vi "Test Base Card Passthrough(Register).vi"(4 "Iterations":u32=50 min=1 max=64, 11 "device":refnum<k21>="SET-2010-Mod2") -> (0 "error out":errorcluster, 1 "Disconnect Timing":T1, 2 "Connect Timing":T1)   [LabVIEW 2020, in "slsc-switch-benchmarks.lvlib"]
uses:
  slsc-switch-benchmarks.lvlib
  Timing Statistics.ctl
  <vilib>/SLSC/Write Register (U64).vi
  <vilib>/SLSC/Initialize Session with Devices.vi
  <vilib>/SLSC/Close Session.vi
  <vilib>/SLSC/SLSC.lvlib
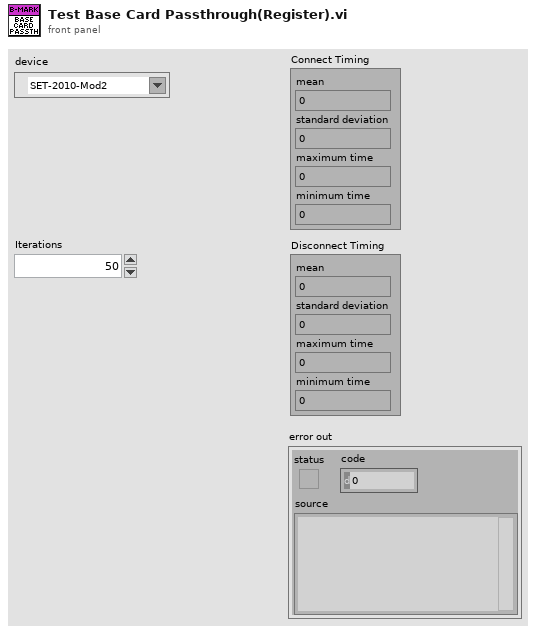
[diagram p1: front panel]
types:
  T1 = typedef "slsc-switch-benchmarks.lvlib/Timing Statistics.ctl" = cluster{"mean":dbl, "standard deviation":dbl, "maximum time":dbl, "minimum time":dbl}
  T2 = cluster{"Connect Time":dbl, "Disconnect Time":dbl}
  T3 = cluster{"Connect Time":dbl, "Disconnect Time":dbl}[]
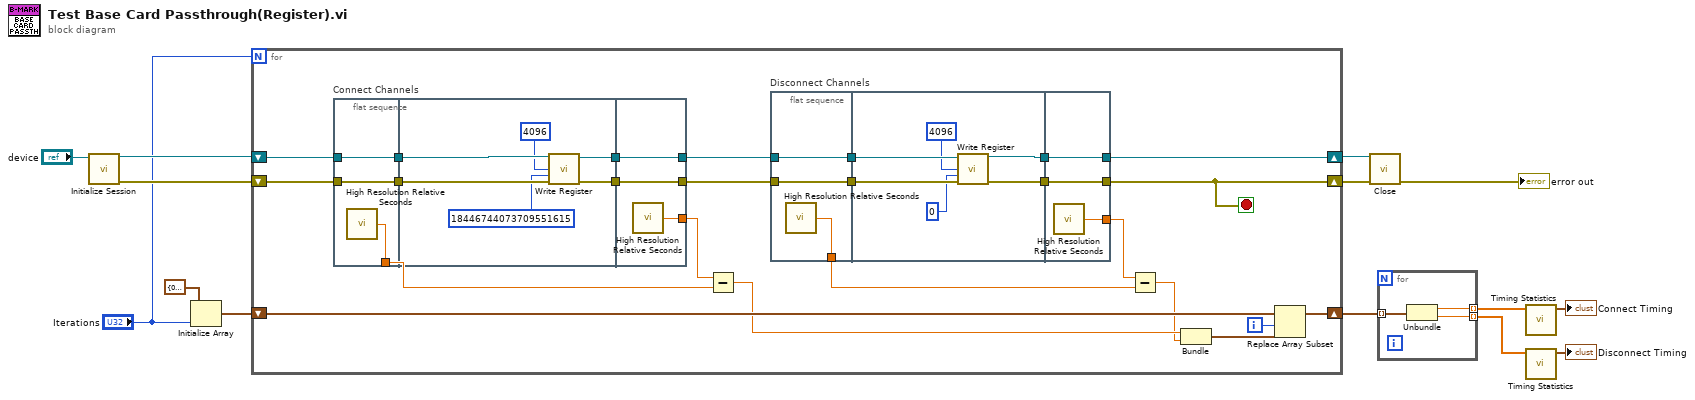
[diagram p0: block diagram]
diagram:
  n1 = call-poly <vilib>:"Initialize Session.vi"("devices"="device") -> ("session out"=w8:refnum<k21>, "error out"=w7:errorcluster)  [unwired: 13 in]
  n2 = Initialize Array(T2 {"Connect Time"=0.0, "Disconnect Time"=0.0}, "Iterations") -> (w14:T3)
  n3 = for {
    N: "Iterations" -> [_]
    shift-right: [w34] -> w5
    shift-left: w8 -> [w38]
    shift-right: [w21] -> w6
    shift-left: w7 -> [w37]
    shift-right: [w18] -> w13
    shift-left: w14 -> [w19]
    i -> [w20]
    stop <- w21 stop-if-true
    n4 = flat-sequence "Connect Channels" {
      tunnel: w37 -> [w52]
      tunnel: w38 -> [w53]
      tunnel: [w53] -> w31
      tunnel: [w52] -> w30
      tunnel: [w51] -> w28
      tunnel: [w56] -> w33
      tunnel: [w57] -> w32
      tunnel: w31 -> [w59]
      tunnel: w30 -> [w58]
      tunnel: [w61] -> w35
      tunnel: [w62] -> w36
      tunnel: w33 -> [w62]
      tunnel: w32 -> [w61]
      tunnel: [w60] -> w29
      frame #0 {
        n5 = call <vilib>:"High Resolution Relative Seconds.vi"() -> ("relative seconds"=w51:dbl)
      }
      frame #1 {
        n6 = call-poly <vilib>:"Write Register.vi"("session in"=w59, "register address"=u32 4096, "data"=u64 18446744073709551615, "error in (no error)"=w58) -> ("session out"=w56:refnum<k21>, "error out"=w57:errorcluster)  [unwired: 8 in, 2 out]
      }
      frame #2 {
        n7 = call <vilib>:"High Resolution Relative Seconds.vi"() -> ("relative seconds"=w60:dbl)
      }
    }
    n8 = Subtract(x=w29, y=w28) -> (x-y=w17:dbl)
    n9 = flat-sequence "Disconnect Channels" {
      tunnel: w35 -> [w40]
      tunnel: w36 -> [w41]
      tunnel: [w41] -> w27
      tunnel: [w40] -> w26
      tunnel: [w39] -> w22
      tunnel: w27 -> [w47]
      tunnel: w26 -> [w46]
      tunnel: [w43] -> w25
      tunnel: [w42] -> w24
      tunnel: [w49] -> w34
      tunnel: [w50] -> w21
      tunnel: w25 -> [w50]
      tunnel: w24 -> [w49]
      tunnel: [w48] -> w23
      frame #0 {
        n10 = call <vilib>:"High Resolution Relative Seconds.vi"() -> ("relative seconds"=w39:dbl)
      }
      frame #1 {
        n11 = call-poly <vilib>:"Write Register.vi"("session in"=w47, "register address"=u32 4096, "data"=u64 0, "error in (no error)"=w46) -> ("session out"=w42:refnum<k21>, "error out"=w43:errorcluster)  [unwired: 8 in, 2 out]
      }
      frame #2 {
        n12 = call <vilib>:"High Resolution Relative Seconds.vi"() -> ("relative seconds"=w48:dbl)
      }
    }
    n13 = Subtract(x=w23, y=w22) -> (x-y=w16:dbl)
    n14 = Bundle(w17, w16) -> (w15:cluster{dbl, dbl})  [unwired: 1 in]
    n15 = Replace Array Subset(array=w19, new element=w15, index=w20) -> (w18:T3)
  }
  n16 = call-poly <vilib>:"Close.vi"("session in"=w5, "error in (no error)"=w6) -> ("error out"=→"error out":errorcluster)  [unwired: 13 in]
  n17 = for {
    tunnel: w13 -> [w65] mode=indexing
    tunnel: [w64] -> w12 mode=indexing
    tunnel: [w63] -> w11 mode=indexing
    n18 = Unbundle(w65) -> ("Connect Time"=w64:dbl, "Disconnect Time"=w63:dbl)
  }
  n19 = call "Timing Statistics.vi"("Execution Speeds"=w12) -> ("Timing Statistics"=→"Connect Timing":T1)  [unwired: 10 in]
  n20 = call "Timing Statistics.vi"("Execution Speeds"=w11) -> ("Timing Statistics"=→"Disconnect Timing":T1)  [unwired: 10 in]
